vi "mes~产品加工参数采集.vi"(8 "error in (no error)":errorcluster caption="错误输入（无错误）", 9 "采集项":string[](array[string])) -> (0 "error out":errorcluster caption="错误输出", 1 "ErrorMessage":string, 2 "加工参数采集成功":bool)   [LabVIEW 2020]
uses:
  Global.vi
  <vilib>/addons/_JKI.lib/Serialization/JSON/JKI JSON Serialization.lvlib
panel:
  in  "Headers":string[][](array[string])=[["Content-Type", "application/json"]]
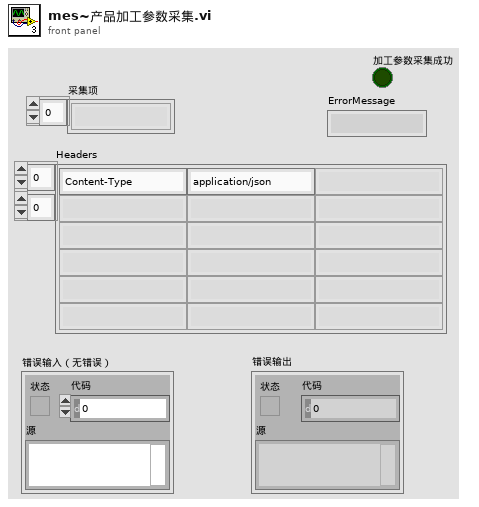
[diagram p1: front panel]
types:
  T1 = cluster{"traceCode":string, "fields":string[], "datas":string}
  T2 = cluster{"接口地址(URL)":string, "用户登录":string, "产品进站":string, "参数采集":string, "产品出站":string, "设备状态":string, "设备编号(equipNum)":string, "站点名称(siteCode)":string, "生产类型(productType)":string, "追溯编号(traceCode)":string}
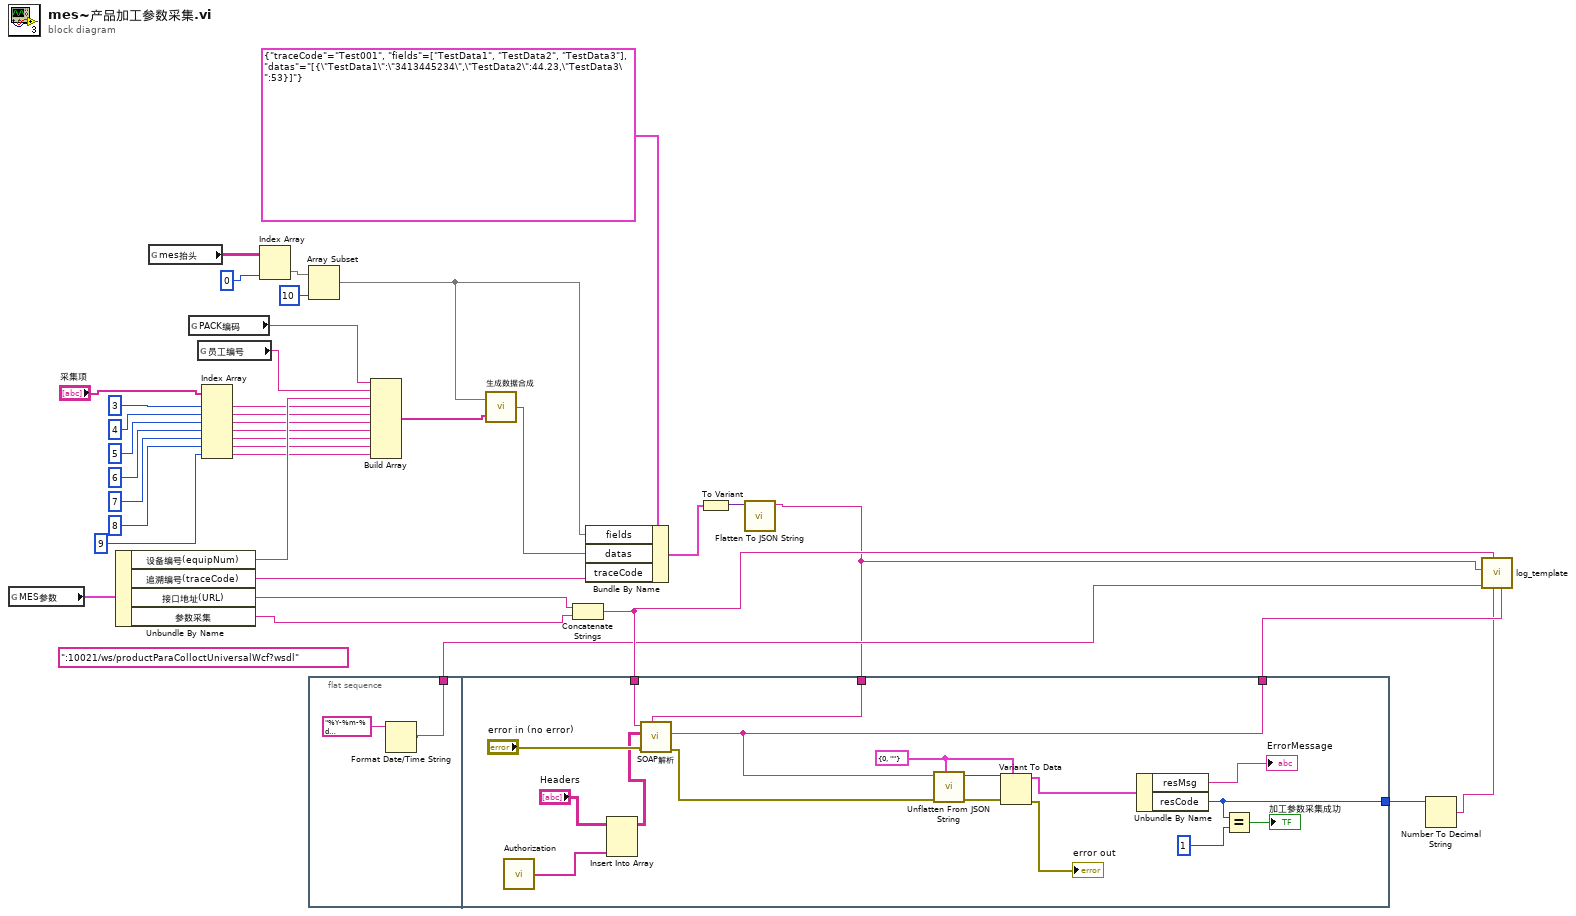
[diagram p0: block diagram]
diagram:
  (unwired) ":10021/ws/productParaColloctUniversalWcf?wsdl"
  n1 = global read "Global.vi" "MES参数"() -> (w37:T2)
  n2 = Unbundle By Name(w37) -> ("设备编号(equipNum)"=w12:string, "追溯编号(traceCode)"=w20:string, "接口地址(URL)"=w3:string, "参数采集"=w30:string)
  n3 = global read "Global.vi" "mes抬头"() -> (w19:string[][])
  n4 = global read "Global.vi" "PACK编码"() -> (w14:string)
  n5 = global read "Global.vi" "员工编号"() -> (w13:string)
  n6 = Index Array(array="采集项", index #1=3 ("索引"), index #2=4 ("索引"), index #3=5 ("索引"), index #4=6 ("索引"), index #5=7 ("索引"), index #6=8 ("索引"), index #7=9 ("索引")) -> (element #1=w11:string, element #2=w10:string, element #3=w9:string, element #4=w8:string, element #5=w7:string, element #6=w6:string, element #7=w1:string)
  n7 = Index Array(array=w19, index (col)=0 ("禁用的索引 (列)")) -> (element=w17:string[])  [unwired: 1 in]
  n8 = Array Subset(array=w17, length=10) -> (w15:string[])  [unwired: 1 in]
  n9 = flat-sequence {
    tunnel: [w39] -> w27
    tunnel: w22 -> [w54]
    tunnel: w28 -> [w55]
    tunnel: [w41] -> w26
    tunnel: [w52] -> w25
    frame #0 {
      n10 = Format Date/Time String(time format string (%c)="%Y-%m-%d %H:%M:%S%3u-->" ("EndTime")) -> (date/time string=w39:string)  [unwired: 2 in]
    }
    frame #1 {
      w46 = cluster{"resCode":i32, "resMsg":string} {"resCode"=0, "resMsg"=""} ("用户登录ctl")
      n11 = call "Authorization.vi"() -> ("Authorization"=w51:string[])
      n12 = Insert Into Array(array="Headers", new element=w51) -> (w49:string[][])  [unwired: 2 in]
      n13 = call "SOAP解析.vi"("DATA"=w54, "错误输入（无错误）"="error in (no error)", "Headers"=w49, "URL"=w55) -> ("错误输出"=w44:errorcluster, "body"=w41:string)  [unwired: 5 in, 1 out]
      n14 = call <vilib>:"Unflatten From JSON String.vi"("Type and Defaults"=w46, "error in (no error)"=w44, "JSON String"=w41) -> ("error out"=w48:errorcluster, "Variant"=w47:variant)  [unwired: 7 in]
      n15 = Variant To Data(error in=w48, type=w46, Variant=w47) -> (data=w43:cluster{"resCode":i32, "resMsg":string}, error out=→"error out":errorcluster)
      n16 = Unbundle By Name(w43) -> ("resMsg"=→"ErrorMessage":string, "resCode"=w52:i32)
      n17 = Equal?(x=w52, y=1) -> (x = y?=→"加工参数采集成功":bool)
    }
  }
  n18 = Build Array(w14, w13, w12, w11, w10, w9, w8, w7, w6, w1) -> (w5:string[])
  n19 = call "生成数据合成.vi"("datas"=w5, "fields"=w15) -> ("fields-datas"=w4:string)
  n20 = Concatenate Strings(w3, w30) -> (w28:string)
  n21 = Bundle By Name(cluster=T1 {"traceCode"="Test001", "fields"=["TestData1", "TestData2", "TestData3"], "datas"="[{\"TestData1\":\"3413445234\",\"TestData2\":44.23,\"TestData3\":53}]"} ("用户登录ctl"), "fields"=w15, "datas"=w4, "traceCode"=w20) -> (w38:T1)
  n22 = To Variant(anything=w38) -> (Variant=w23:variant)
  n23 = call <vilib>:"Flatten To JSON String.vi"("Variant"=w23) -> ("JSON String"=w22:string)  [unwired: 9 in, 1 out]
  n24 = Number To Decimal String(number=w25) -> (decimal integer string=w24:string)  [unwired: 1 in]
  n25 = call "log_template.vi"("接收报文"=w26, "a:Success"=w24, "URL"=w28, "StartTime"=w27, "发送报文"=w22) -> ()  [unwired: 7 in]
